vi "Muestreo.vi"() -> ()   [LabVIEW 2026]
panel:
  in  "Min_max_pwm":i32[][](array[numeric])
  in  "Min_max_pulsos":i32[][](array[numeric])
  out "Pasos_Por_Grado":i32[](array[numeric])
  in  "Estado_Conexion":u32
  in  "Conador_incorrecto":u32
  in  "Contador_correcto":u32
  in  "Tramas":i32
  in  "V_baud":u32
  in  "V_buf_t":u32
  in  "V_timeout":u32
  in  "Pack_t":i32
  in  "Bytes_at_port":u32
  in  "T_muestreo":dbl
  # "Periodo de muestreo"
  # "Tamaño del paquete completo enviado por la esp32"
  # "Tamaño de cada trama individual enviada"
  # "Número de tramas dentro del paquete en la esp32"
  # "Visa timeout"
  # "Visa buffer size"
  # "Visa baud rate"
  # "Contador_correcto"
  # "Contador_incorrecto"
  # "Estado_conexion"
  # "Pasos por grado de movimiento de la articulación"
  # "[Mín,Max] número de pulsos que se puede mover la articulación"
  # "[Mín,Max] PWM"
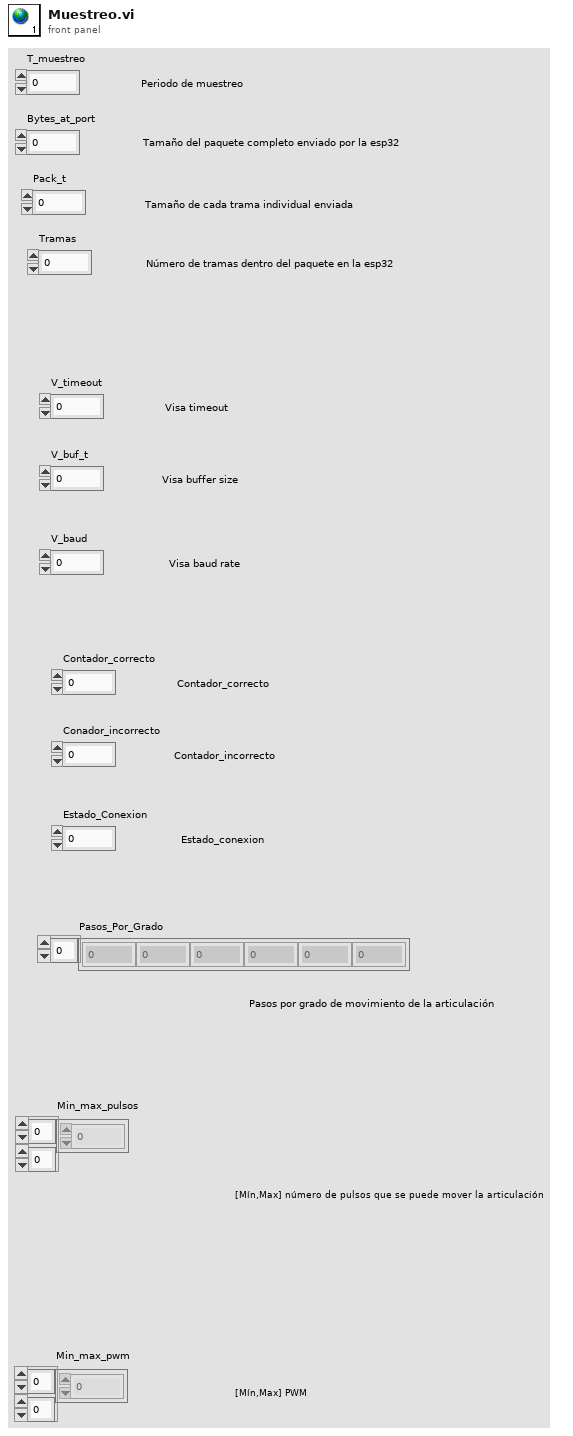
[diagram p1: front panel]
diagram:
